vi "Read Image Information.vi"(8 "error in (no error)":errorcluster, 11 "Save Image in":refnum<class "Save Image.lvclass">) -> (0 "error out":errorcluster, 2 "Image Information":T1, 3 "Save Image out":refnum<class "Save Image.lvclass">)   [LabVIEW 2018, in "Save Image.lvclass"]
uses:
  Save Image.lvclass
  Save Image.lvclass/Save Image.ctl
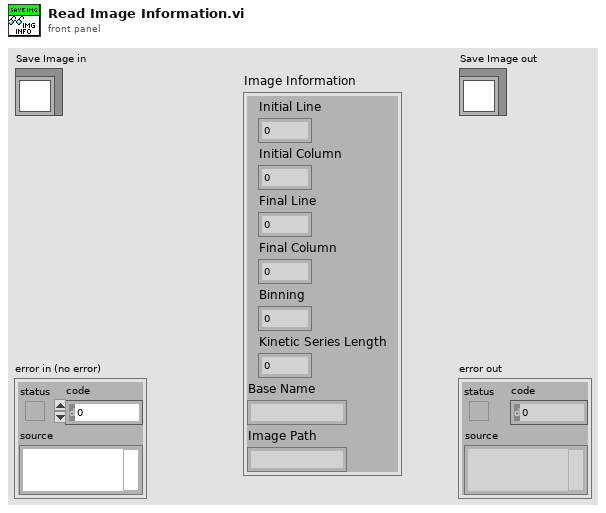
[diagram p1: front panel]
types:
  T1 = cluster{"Initial Line":u16, "Initial Column":u16, "Final Line ":u16, "Final Column":u16, "Binning":u16, "Kinetic Series Length":u16, "Base Name":string, "Image Path":string}
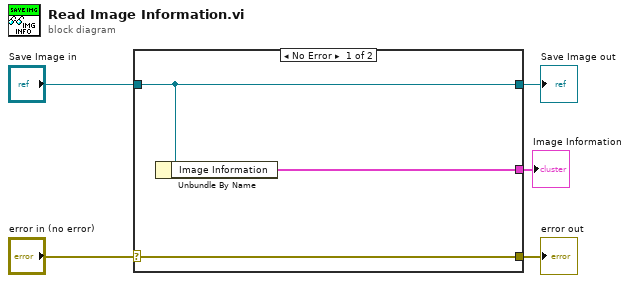
[diagram p0: block diagram]
diagram:
  n1 = case shown="No Error" "error in (no error)" {
    selector: "error in (no error)" -> [w8 w9]
    tunnel: [w8 w9] -> w4
    tunnel: [w7 w10] -> w2
    tunnel: "Save Image in" -> [w7 w10]
    tunnel: [w6 _] -> w1
    frame No Error {
      n2 = Unbundle By Name(w7) -> ("Image Information"=w6:T1)
    }
    frame Error {
    }
  }
  "error out" <- w4
  "Save Image out" <- w2
  "Image Information" <- w1
